vi "Pre-Install Action.vi"(10 "Variant":variant) -> (0 "error out":errorcluster)   [LabVIEW 2014]
uses:
  <vilib>/zip/NI_Unzip.lvlib
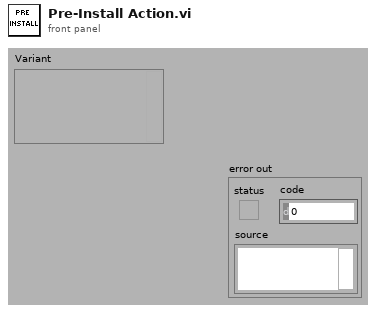
[diagram p1: front panel]
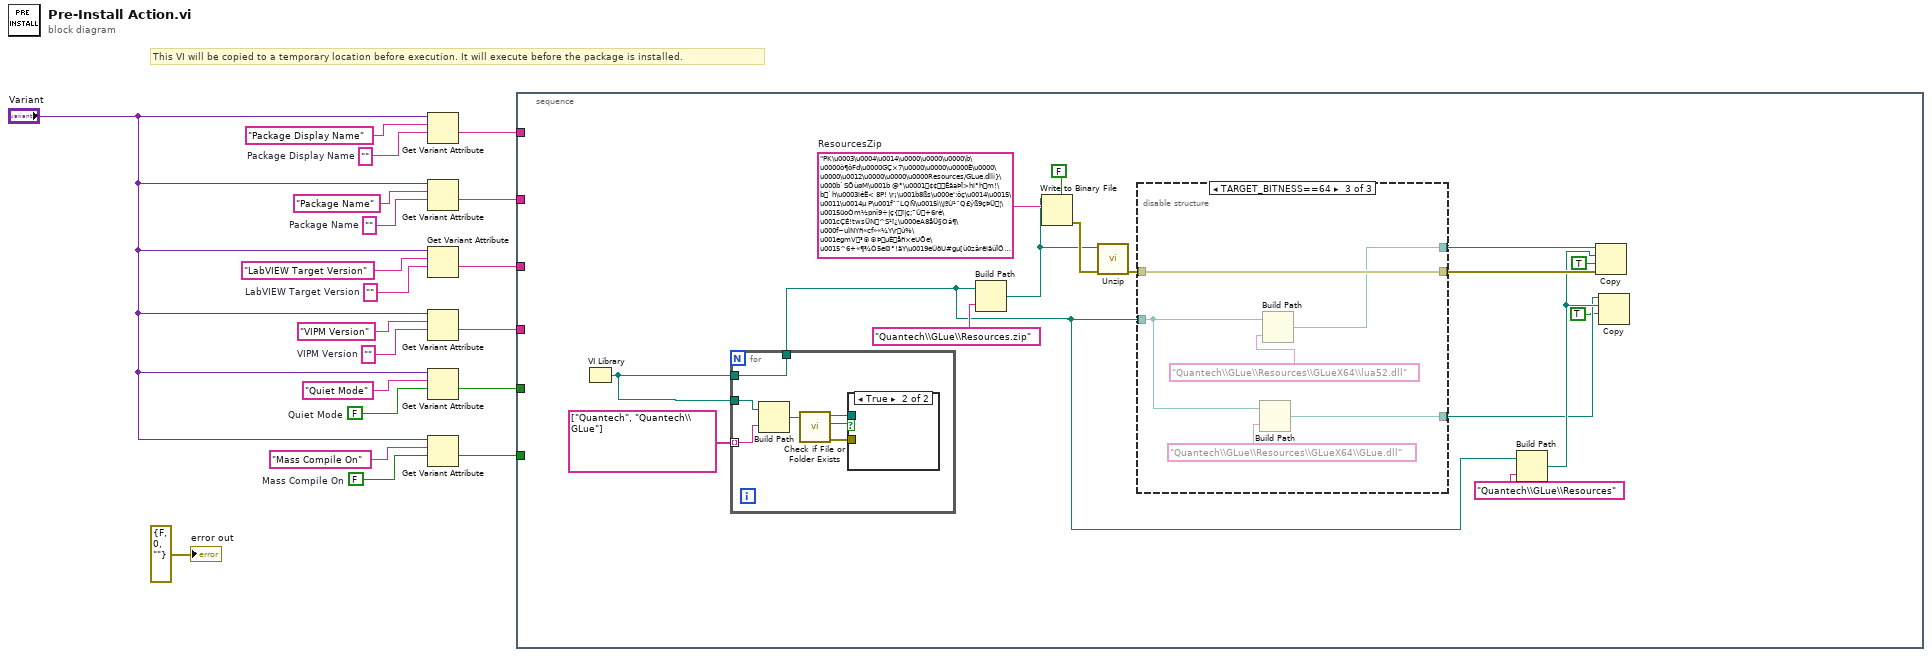
[diagram p0: block diagram]
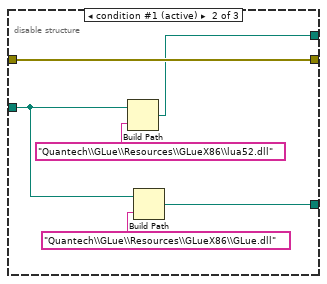
[diagram p3: hidden frame]
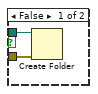
[diagram p4: hidden frame]
diagram:
  w1 = FALSE  # Mass Compile On
  w3 = ""  # Package Display Name
  w10 = FALSE  # Quiet Mode
  w13 = ""  # VIPM Version
  w15 = ""  # LabVIEW Target Version
  w17 = ""  # Package Name
  # "This VI will be copied to a temporary location before execution. It will execute before the package is installed."
  n1 = Get Variant Attribute(Variant="Variant", name="Package Display Name", default value (empty Variant)=w3) -> (value=w9:string)  [unwired: 1 in, 3 out]
  n2 = Get Variant Attribute(Variant="Variant", name="Package Name", default value (empty Variant)=w17) -> (value=w8:string)  [unwired: 1 in, 3 out]
  n3 = Get Variant Attribute(Variant="Variant", name="LabVIEW Target Version", default value (empty Variant)=w15) -> (value=w7:string)  [unwired: 1 in, 3 out]
  n4 = Get Variant Attribute(Variant="Variant", name="VIPM Version", default value (empty Variant)=w13) -> (value=w6:string)  [unwired: 1 in, 3 out]
  n5 = Get Variant Attribute(Variant="Variant", name="Quiet Mode", default value (empty Variant)=w10) -> (value=w5:bool)  [unwired: 1 in, 3 out]
  n6 = Get Variant Attribute(Variant="Variant", name="Mass Compile On", default value (empty Variant)=w1) -> (value=w4:bool)  [unwired: 1 in, 3 out]
  n7 = stacked-sequence {
    tunnel: w9 -> [_]
    tunnel: w8 -> [_]
    tunnel: w7 -> [_]
    tunnel: w6 -> [_]
    tunnel: w5 -> [_]
    tunnel: w4 -> [_]
    frame #0 {
      w36 = "PK\u0003\u0004\u0014\u0000\u0000\u0000\b\u0000ò¶ôFd\u0000GÇ×7\u0000\u0000\u0000Ê\u0000\u0000\u0012\u0000\u0000\u0000Resources/GLue.dllí}\u000b`SÕùøM\u001b @°\u0001¢¢ÊäaÞÏ>hi°hm!\b`h\u0003iéË< 8P! \r¡\u001b8ßs\u000e':ôç\u0014\u0015\u0011\u0014µ P\u001f¨¨LQÑ\u0015ì\\jºÙ¹¨Q£ýß9çÞÜ¦\u0015üoÓm½pnî9÷|ç{ï|ç;¯Û+6ré\u001cÇÉ!twsÜN^S¹ï¿\u000eA8åÜ§Oá¶\u000f~uÌNYñ«cf»«¼Y\rú%\u001egmV³®®ÞµÈåñ×eUÕe\u0015^6+«¶¾Ò5eØ°!ãY\u0019eÚõU#gµ[ù0zârëiäùÏÖ\u0011ð{Êk3­gßë­ä÷:ö»üWU¸\u0011§©ÔÎqÅ²Ü«ÿààÓÚ¸´1CeC8n\u0003DrE\f¨ lfOøÆq\u00038\u0019Ià9üÓ§tnê\u0000\u0002¤bÀªD1Ü\u0003\u001c·{ \u0015Ê\u0004'O!´.)(ÞÑ' cþòA¹Å}¼âs5úà7\u001ab\u0004!¯Iø³8îê)J§ÏÉqN¡4¼\u001b¥ù¦Âÿ)4\u001bu\u001aÜ¶AÈäxYóµL©¢\u0019\u001bAvD!\u0010çö\u0014ù<^O\u0005ÇdÒ\u0006\u0001eµ³G¾©S<®zÈ¸\u0001ª\u000beÅ)!<×#_A\u001f¢è¿Nâ:WÇ\u0003^ëùáö0(YÇÅÃÍS\t·\u000fæÂ-<\u0015n\u0015WÂíÃ³áö.TMGáÅpËVÜñu\u0011Ü\u001cZ¸\u001dº\u0014nÏ¬Û\u0003Ùp[mÛËàöÔt¸\u0015Àí¯:¸mÖÚ1k\nÜî¹\u0002n?+[;´Ëßzàö4ÔxÇý..."  # ResourcesZip
      n8 = VI Library() -> (path=w30:path)
      n9 = for {
        tunnel: string[] ["Quantech", "Quantech\\GLue"] -> [w54] mode=indexing
        tunnel: w30 -> [w55]
        tunnel: w30 -> [w49]
        tunnel: [w49] -> w24
        n10 = Build Path(base path=w55, name or relative path=w54) -> (appended path=w53:path)
        n11 = call <vilib>:"Check if File or Folder Exists.vi"("path"=w53) -> ("error out"=w50:errorcluster, "file or folder exists?"=w52:bool, "dup path"=w51:path)  [unwired: 8 in]
        n12 = case shown="True" w52 {
          tunnel: w51 -> [w57 _]
          tunnel: w50 -> [w56 _]
          frame False {
            n13 = Create Folder(path (use dialog)=w57, error in=w56) -> ()  [unwired: 1 in, 3 out]
          }
          frame True {
          }
        }
      }
      n14 = Build Path(base path=w24, name or relative path="Quantech\\GLue\\Resources.zip") -> (appended path=w31:path)
      n15 = Write to Binary File(file (use dialog)=w31, data=w36, 5:FALSE ("prepend array or string size? (T)")) -> (error out=w34:errorcluster)  [unwired: 3 in, 2 out]
      n16 = call <vilib>:"Unzip.vi"("error in (no error)"=w34, "Zip file"=w31) -> ("error out"=w29:errorcluster)  [unwired: 7 in, 2 out]
      n17 = disable-structure shown="TARGET_BITNESS==64" {
        disable-tunnel: w29 -> [_ w42 w48]
        disable-tunnel: w24 -> [_ w38 w44]
        disable-tunnel: [_ w42 w48] -> w28
        disable-tunnel: [_ w40 w47] -> w26
        disable-tunnel: [_ w37 w43] -> w22
        frame condition #0 {
        }
        frame condition #1 (active) {
          n18 = Build Path(base path=w38, name or relative path="Quantech\\GLue\\Resources\\GLueX86\\lua52.dll") -> (appended path=w40:path)
          n19 = Build Path(base path=w38, name or relative path="Quantech\\GLue\\Resources\\GLueX86\\GLue.dll") -> (appended path=w37:path)
        }
        frame condition #2 {
          n20 = Build Path(base path=w44, name or relative path="Quantech\\GLue\\Resources\\GLueX64\\GLue.dll") -> (appended path=w43:path)
          n21 = Build Path(base path=w44, name or relative path="Quantech\\GLue\\Resources\\GLueX64\\lua52.dll") -> (appended path=w47:path)
        }
      }
      n22 = Build Path(base path=w24, name or relative path="Quantech\\GLue\\Resources") -> (appended path=w23:path)
      n23 = Copy(8:w28, 9:TRUE ("overwrite (F)"), 10:w23, 11:w26) -> ()  [unwired: 1 in, 3 out]
      n24 = Copy(9:TRUE ("overwrite (F)"), 10:w23, 11:w22) -> ()  [unwired: 2 in, 3 out]
    }
  }
  "error out" <- errorcluster {"status"=FALSE, "code"=0, "source"=""} ("error out")
